vi "Init.vi"(8 "error in (no error)":errorcluster) -> (0 "error out":errorcluster, 3 "Mock Filter out":refnum<class "Mock Filter.lvclass">)   [LabVIEW 2020, in "Mock Filter.lvclass"]
uses:
  Mock Filter.lvclass
  Mock Filter.lvclass/Mock Filter.ctl
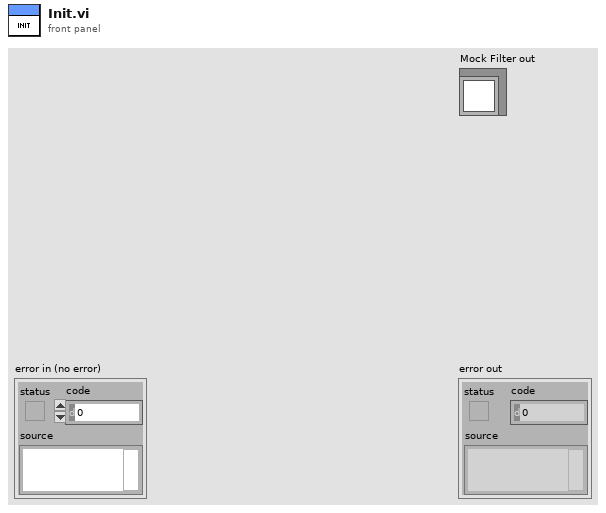
[diagram p1: front panel]
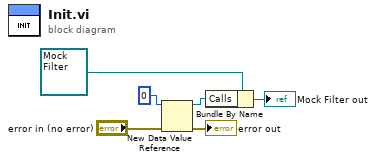
[diagram p0: block diagram]
diagram:
  n1 = New Data Value Reference(data value=0, error in="error in (no error)") -> (data value reference=w3:refnum<data-value>, error out=→"error out":errorcluster)
  n2 = Bundle By Name(cluster=refnum<class "Mock Filter.lvclass"> refnum ("Mock Filter in"), "Calls"=w3) -> (→"Mock Filter out":refnum<class "Mock Filter.lvclass">)
